vi "Crop Image.vi"(0 "Image Src":T1, 2 "Image Refnum":refnum<vi>, 11 "Error in (no error)":errorcluster) -> (4 "Cropped Image":T1, 15 "Error in (no error)":errorcluster)   [LabVIEW 2021]
uses:
  <vilib>/vision/NI_Vision_Development_Module.lvlib
  <resource>/objmgr/IMAQImage.rc
  <vilib>/vision/Image Controls.llb/IMAQ Image.ctl
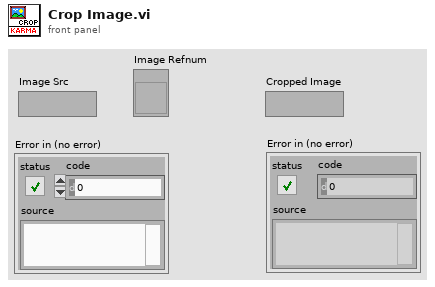
[diagram p1: front panel]
types:
  T1 = typedef "IMAQ Image.ctl" = refnum<image>
  T2 = typedef "Image Type" = u32
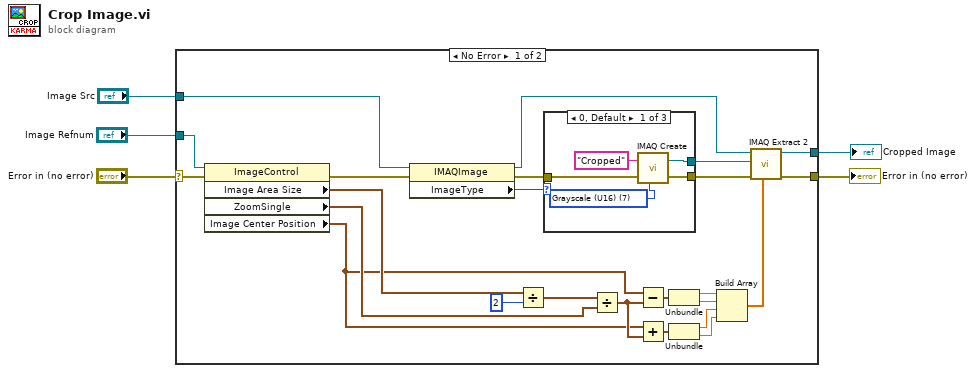
[diagram p0: block diagram]
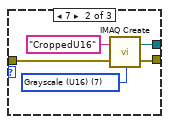
[diagram p2: hidden frame]
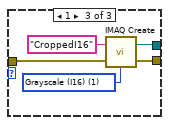
[diagram p3: hidden frame]
diagram:
  n1 = case shown="No Error" "Error in (no error)" {
    selector: "Error in (no error)" -> [w6 w46]
    tunnel: "Image Refnum" -> [w15 _]
    tunnel: "Image Src" -> [w14 w45]
    tunnel: [w8 w45] -> w3
    tunnel: [w7 w46] -> w2
    frame No Error {
      n2 = property on="Property Node" class="ImageControl"(reference=w15, error in=w6) -> (error out=w11:errorcluster, "Image Area Size"=w28:cluster{"Width":u32, "Height":u32}, "ZoomSingle"=w27:cluster{"X":sgl, "Y":sgl}, "Image Center Position"=w19:cluster{"X":u32, "Y":u32})  [unwired: 1 out]
      n3 = property class="IMAQImage"(reference=w14, error in=w11) -> (reference out=w13:T1, error out=w10:errorcluster, "ImageType"=w12:u32)
      n4 = Divide(x=w28, y=2) -> (x/y=w18:cluster{"Width":dbl, "Height":dbl})
      n5 = case shown="0, Default" w12 {
        tunnel: [w31 w37 w42] -> w16
        tunnel: w10 -> [w30 w36 w41]
        tunnel: [w32 w35 w40] -> w9
        frame 0, Default {
          w33 = T2 7 items=["Grayscale (U8)", "Grayscale (I16)", "Grayscale (SGL)", "Complex (CSG)", "RGB (U32)", "HSL (U32)", "RGB (U64)", "Grayscale (U16)"] ("Image Type")
          n6 = call "IMAQ Create"("Image Name"="Cropped", "Image Type"=w33, "error in (no error)"=w30) -> ("New Image"=w31:T1, "error out"=w32:errorcluster)  [unwired: 2 in]
        }
        frame 7 {
          w38 = T2 7 items=["Grayscale (U8)", "Grayscale (I16)", "Grayscale (SGL)", "Complex (CSG)", "RGB (U32)", "HSL (U32)", "RGB (U64)", "Grayscale (U16)"] ("Image Type")
          n7 = call "IMAQ Create"("Image Name"="CroppedU16", "Image Type"=w38, "error in (no error)"=w36) -> ("New Image"=w37:T1, "error out"=w35:errorcluster)  [unwired: 2 in]
        }
        frame 1 {
          w43 = T2 1 items=["Grayscale (U8)", "Grayscale (I16)", "Grayscale (SGL)", "Complex (CSG)", "RGB (U32)", "HSL (U32)", "RGB (U64)", "Grayscale (U16)"] ("Image Type")
          n8 = call "IMAQ Create"("Image Name"="CroppedI16", "Image Type"=w43, "error in (no error)"=w41) -> ("New Image"=w42:T1, "error out"=w40:errorcluster)  [unwired: 2 in]
        }
      }
      n9 = Divide(x=w18, y=w27) -> (x/y=w20:cluster{dbl, dbl})
      n10 = Subtract(x=w19, y=w20) -> (x-y=w21:cluster{dbl, dbl})
      n11 = Add(x=w19, y=w20) -> (x+y=w24:cluster{dbl, dbl})
      n12 = Unbundle(w21) -> (w22:dbl, w23:dbl)
      n13 = Unbundle(w24) -> (w25:dbl, w26:dbl)
      n14 = Build Array(w22, w23, w25, w26) -> (w29:dbl[])
      n15 = call "IMAQ Extract 2"("Optional Rectangle"=w29, "error in (no error)"=w9, "Image Dst"=w16, "Image Src"=w13) -> ("error out"=w7:errorcluster, "Image Dst Out"=w8:T1)  [unwired: 6 in]
    }
    frame Error {
    }
  }
  "Cropped Image" <- w3
  "Error in (no error)" <- w2
